vi "STAGE+mono+counter_edit25.vi"() -> ()   [LabVIEW 2017]
panel:
  out "Timeout":bool
  out "PROGRESS":u8(slide) max=10 step=10 scale=0.0..1.0
  in  "?":enum32{"Scan Data", "Scans", "RT Data"}(tab)
  out "Spectrum":cluster{dbl[], dbl[]}(graph)
  out "Decay":cluster{dbl[], dbl[]}[](graph)
  in  "Collect Data!":bool
  out "Waveform Graph":waveform(dbl)[](graph)
  out "?":i32(knob) scale=0.0..1000000.0
  out "Photon Counts":dbl
  in  "Wavelength":dbl
  in  "Show Real Time Data":bool
  in  "?":enum32{"DELAY", "COUNTER", "MONO", "PLOT"}(tab)
  in  "Data File Path":path
  out "Final time [ps]":dbl
  out "Current time [ps]":dbl
  out "Initial time [ps]":dbl
  in  "Set this as t0":bool
  in  "Axis":i32=1
  in  "Motor ON":bool
  in  "Motor OFF":bool
  out "Current Position [mm]":dbl
  out "Final Position [mm]":dbl
  in  "Data Points":i32=100
  out "Current Point":i32
  in  "Step Size [um]":i32=10
  in  "Target [mm]":dbl format="%.3f"
  in  "Move":bool
  out "Initial position [mm]":dbl
  in  "GPIB address":string="23"
  in  "Count Mode":u16(ring) items=["A,B for Preset T", "A-B for Preset T", "A+B for Preset T", "A for Preset B"]
  in  "Trigger mode":u16(ring) items=["10 MHz"=0, "Input 2"=2, "Input T"=3]
  in  "Channel A Input":u16(ring)=1 items=["10 MHz", "Input 1"]
  in  "Channel B Input":u16(ring)=2 items=["Input 1"=1, "Input 2"=2]
  in  "Number of Measurements\n to take at one point/ Number of Periods":u16=1 min=1 max=2000 step=1
  in  "Time between measurements\n at one point (s)/Dwell Time":dbl=0.002 min=0.002 max=60.0 step=0.001
  in  "gate mode (CW:0)":i16(slide) scale=0.0..2.0 scale format="%.2f"
  out "Counts":i32
  in  "Integrating time \nin 10^-7 sec":dbl=10000000.0
  in  "Discriminator Level (mV)":dbl min=-300.0 max=300.0 step=0.2
  in  "Discriminator Slope":bool
  in  "Channel":i16 min=0 max=2 step=1
  out "Grating #":dbl
  out "Blaze angle":dbl
  out "Grooves/mm":dbl
  out "Mono port":T1(ring)
  out "Time delay":u32=450000 min=1
  in  "Step size":dbl=10.0 min=0.0
  in  "Scan to":i32=4000
  in  "Scan from":i32=2600
  out "Current wavelength":dbl
  in  "?":bool
  in  "NEW UNIT":T2(ring)
  in  "Array":dbl[](array[numeric])
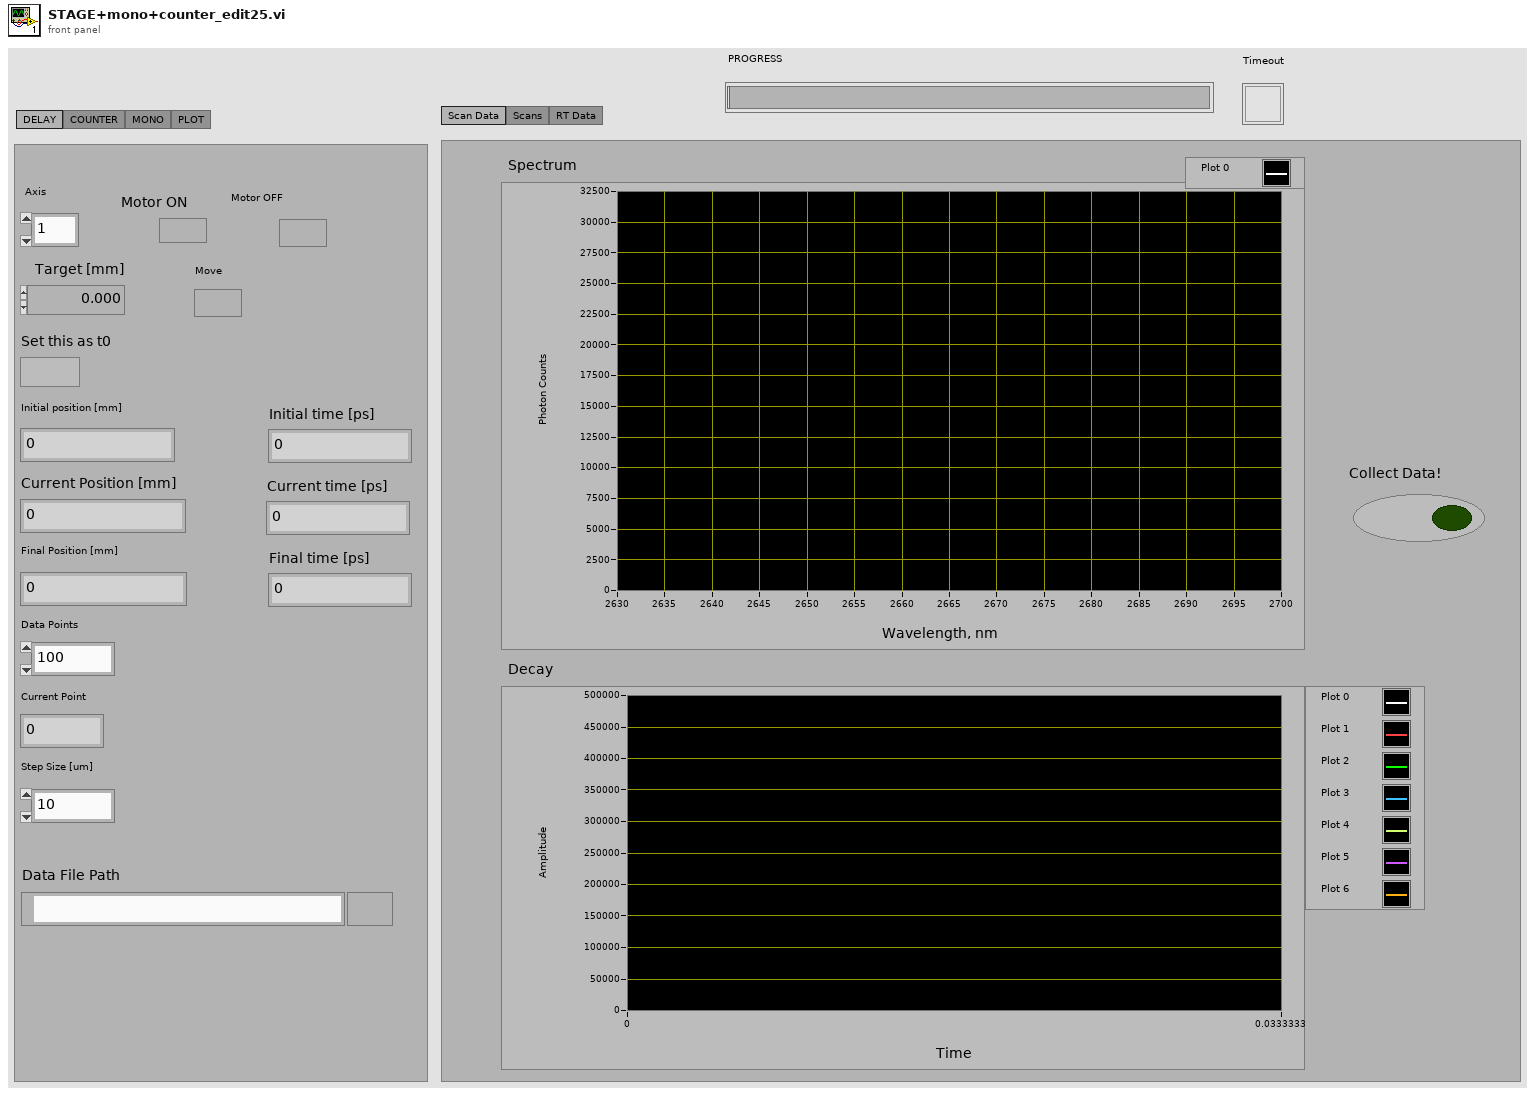
[diagram p1: front panel]
types:
  T1 = enum8{"COM 1", "COM 2", "COM 3", "COM 4", "COM 5", "COM 6", "COM 7", "COM 8", "COM 9"}
  T2 = enum16{"centi-Microns", " Nanometers", "   Angstroms"}
  T3 = cluster{"input XON/XOFF":bool, "input HW Handshake":bool, "input alt HW HShk":bool, "output XON/XOFF":bool, "output HW Handshake":bool, "output alt HW HShk":bool, "XOFF byte":u8, "XON byte":u8, "parity error byte":u16}
  T4 = enum16{"no parity", "odd parity", "even parity", "mark parity", "space parity"}
  T5 = enum16{"open", "replace", "create", "open or create", "replace or create", "replace or create with confirmation"}
  T6 = typedef "NI_Matrix.lvlib/RealMatrix.ctl" = dbl[][]
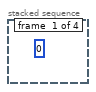
[diagram p2: hidden frame]
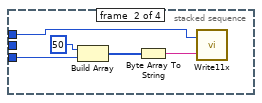
[diagram p3: hidden frame]
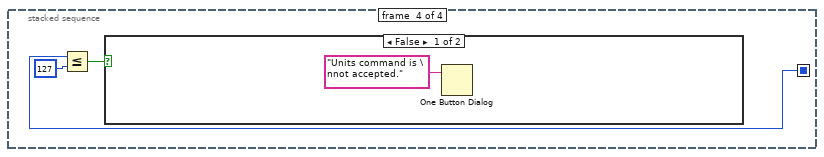
[diagram p4: hidden frame]
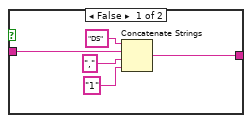
[diagram p7: hidden frame]
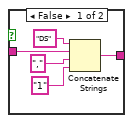
[diagram p9: hidden frame]
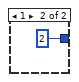
[diagram p13: hidden frame]
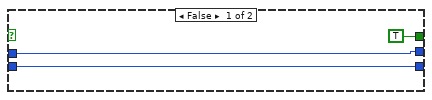
[diagram p14: hidden frame]
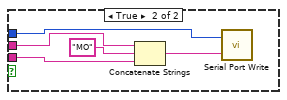
[diagram p15: hidden frame]
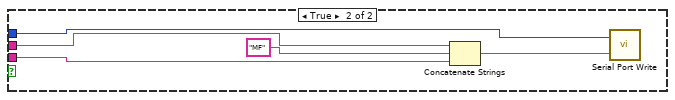
[diagram p16: hidden frame]
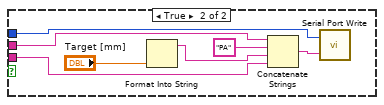
[diagram p17: hidden frame]
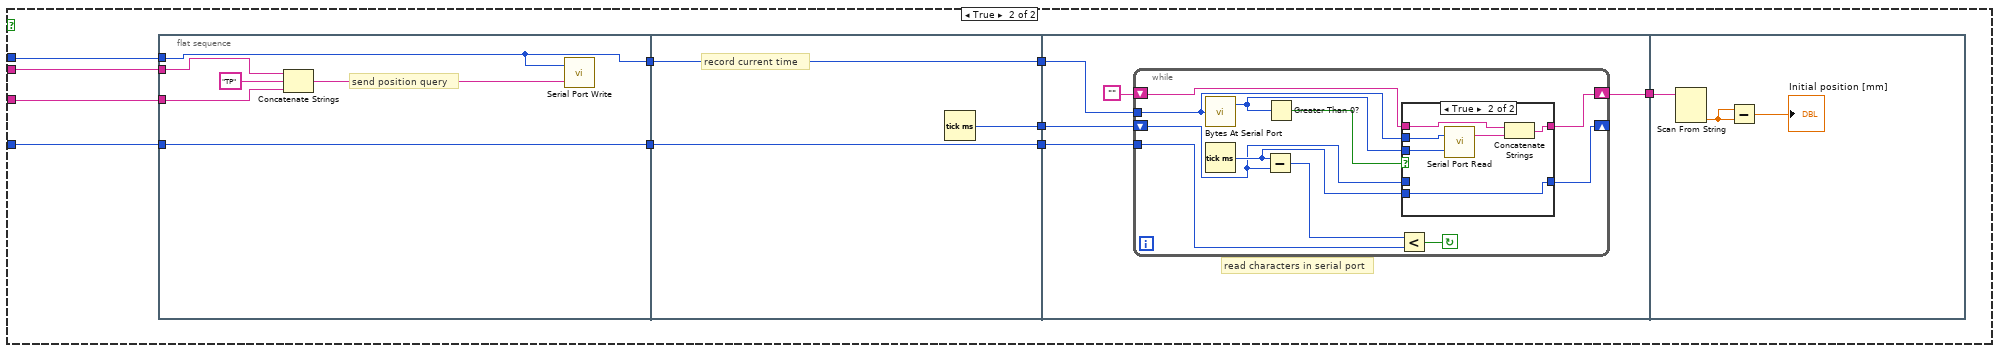
[diagram p18: hidden frame]
diagram:
  w29 = u32 19200  # baud rate
  w28 = u16 8  # data bits
  w27 = enum16{"1 bit", "1.5 bits", "2 bits"}."1 bit"  # stop bits
  w31 = T4."no parity"  # parity
  w9 = 4  # 0=COM1 so n=COM(n+1)
  w30 = u16 1024  # buffer size
  n1 = flat-sequence {
    tunnel: [w34] -> w1
    tunnel: [w33] -> w2
    frame #0 {
      n2 = call "CM Com Read ini.vi"() -> ("Mono port"=w33:T1, "time delay1"=w34:u32)  [unwired: 7 in]
    }
  }
  n3 = stacked-sequence {
    seq-local: [_ _ w42 _] -> [_ _ _ w49]
    tunnel: "NEW UNIT" -> [_ w36 _ _]
    tunnel: w1 -> [_ w35 w40 _]
    tunnel: w2 -> [_ _ w41 _]
    frame #0 {
      (unwired) u8 0
    }
    frame #1 {
      n4 = Build Array(u8 50, w36) -> (w38:u16[])
      n5 = Byte Array To String(unsigned byte array=w38) -> (string=w37:string)
      n6 = call "Write11x.vi"("string to write"=w37, "port number"=w35) -> ()  [unwired: 1 out]
    }
    frame #2 {
      n7 = call "Read11x.vi"("response size"=2, "timeout count"=w41, "port number"=w40) -> ("rcv index"=w43:u8[])  [unwired: 2 out]
      n8 = Index Array(array=w43, index=1) -> ()  [unwired: 1 out]
      n9 = Index Array(array=w43, index=0) -> (element=w42:u8)
    }
    frame #3 {
      n10 = Less Or Equal?(x=w49, y=127) -> (x <= y?=w47:bool)
      n11 = case shown="False" w47 {
        frame False {
          n12 = One Button Dialog(message="Units command is \nnot accepted.") -> ()  [unwired: 1 in, 1 out]
        }
        frame True {
        }
      }
    }
  }
  n13 = call "CM Serial Port Setup.vi"("COM port"=w2, "time delay"=w1) -> ("time delay1"=w19:u32, "DK port Out"=w20:T1, "error code"=w22:i32)  [unwired: 7 in]
  n14 = Equal To 0?(x=w22) -> (x = 0?=w21:bool)
  n15 = case shown="True" w21 {
    tunnel: w20 -> [w53 w56]
    tunnel: w19 -> [w52 w55]
    tunnel: [w53 w56] -> w6
    tunnel: [w52 w55] -> w5
    tunnel: [TRUE FALSE] -> w4
    frame False {
    }
    frame True {
      n16 = call "CM Com Write ini.vi"("time delay1"=w56, "Mono port"=w55) -> ()  [unwired: 7 in]
      n17 = local write "Mono port"(w56) -> ()
      n18 = local write "Time delay"(w55) -> ()
    }
  }
  n19 = call <vilib>:"Serial Port Init.vi"("flow control etc."=T3 {"input XON/XOFF"=FALSE, "input HW Handshake"=FALSE, "input alt HW HShk"=FALSE, "output XON/XOFF"=FALSE, "output HW Handshake"=FALSE, "output alt HW HShk"=FALSE, "XOFF byte"=13, "XON byte"=11, "parity error byte"=0}, "parity"=w31, "buffer size"=w30, "stop bits"=w27, "data bits"=w28, "baud rate"=w29, "port number"=w9) -> ("error code"=w26:i32)
  n20 = Concatenate Strings("\r", "\n") -> (w23:string)
  n21 = while {
    tunnel: w5 -> [w59]
    tunnel: w6 -> [w58]
    stop <- TRUE continue-if-true
    n22 = case shown="True" "?" {
      tunnel: w59 -> [_ w62]
      tunnel: w58 -> [_ w61]
      frame False {
      }
      frame True {
        n23 = Two Button Dialog(message="Do you want to change grating?", 1:"No" ("F button name (\"Cancel\")"), 2:"Yes" ("T button name (\"OK\")")) -> (T button?=w63:bool)
        n24 = case shown="True" w63 {
          tunnel: w62 -> [_ w68]
          tunnel: w61 -> [_ w67]
          frame False {
          }
          frame True {
            n25 = Two Button Dialog(message="Disable voltage from PMT", 1:"Do not swich grating" ("F button name (\"Cancel\")"), 2:"Done" ("T button name (\"OK\")")) -> (T button?=w69:bool)
            n26 = case shown="True" w69 {
              tunnel: w68 -> [_ w81]
              tunnel: w67 -> [_ w80]
              frame False {
              }
              frame True {
                n27 = flat-sequence {
                  tunnel: w81 -> [w85]
                  tunnel: [w85] -> w75
                  tunnel: w80 -> [w84]
                  tunnel: [w84] -> w74
                  tunnel: [w82] -> w73
                  tunnel: w75 -> [w90]
                  tunnel: [w90] -> w78
                  tunnel: w74 -> [w91]
                  tunnel: [w91] -> w77
                  tunnel: w73 -> [w89]
                  tunnel: [w89] -> w76
                  tunnel: w78 -> [w95]
                  tunnel: w77 -> [w96]
                  tunnel: [w94] -> w79
                  tunnel: w76 -> [w94]
                  frame #0 {
                    n28 = local read "Grating #"() -> (w83:dbl)
                    n29 = case shown="2, Default" w83 {
                      tunnel: [1 2] -> w82
                      frame 2, Default {
                      }
                      frame 1 {
                      }
                    }
                    n30 = call "Select11x2.vi"("time delay"=w85, "NEW GRT?"=w82, "port number"=w84) -> ()  [unwired: 3 out]
                  }
                  frame #1 {
                    n31 = call "Query11x.vi"("port number"=w91, "QUERY"=u16 2, "time delay"=w90) -> ("STATUS MESSAGE"=w88:u16)  [unwired: 3 out]
                    n32 = local write "Grooves/mm"(w88) -> ()
                  }
                  frame #2 {
                    n33 = Divide(x=w95, y=i16 100 ("device (1)")) -> (x/y=w97:dbl)
                    n34 = call "Query11x.vi"("port number"=w96, "QUERY"=u16 3, "time delay"=w97) -> ("STATUS MESSAGE"=w93:u16)  [unwired: 3 out]
                    n35 = local write "Blaze angle"(w93) -> ()
                  }
                }
                n36 = local write "Grating #"(w79) -> ()
              }
            }
          }
        }
      }
    }
  }
  n37 = while {
    tunnel: w9 -> [w114]
    tunnel: w23 -> [w115]
    tunnel: w26 -> [_]
    tunnel: "Axis" -> [w112]
    stop <- TRUE continue-if-true
    w113 = u32 200  # timeout
    n38 = Format Into String(w112) -> (resulting string=w116:string)  [unwired: 3 in, 1 out]
    n39 = flat-sequence {
      tunnel: w116 -> [w121]
      tunnel: w115 -> [w120]
      tunnel: w114 -> [w122]
      tunnel: w113 -> [w119]
      tunnel: [w121] -> w111
      tunnel: [w120] -> w110
      tunnel: [w122] -> w109
      tunnel: [w119] -> w108
      tunnel: w111 -> [w132]
      tunnel: w110 -> [w131]
      tunnel: w109 -> [w133]
      tunnel: w108 -> [w129]
      tunnel: [w132] -> w107
      tunnel: [w131] -> w106
      tunnel: [w133] -> w105
      tunnel: [w129] -> w104
      tunnel: w107 -> [w142]
      tunnel: w106 -> [w141]
      tunnel: w105 -> [w143]
      tunnel: w104 -> [w139]
      tunnel: [w142] -> w103
      tunnel: [w141] -> w102
      tunnel: [w143] -> w101
      tunnel: [w139] -> w100
      tunnel: w103 -> [w155]
      tunnel: w102 -> [w152]
      tunnel: w101 -> [w154]
      tunnel: w100 -> [w153]
      frame #0 {
        n40 = case shown="False" "Motor ON" {
          tunnel: w122 -> [_ w128]
          tunnel: w121 -> [_ w125]
          tunnel: w120 -> [_ w124]
          frame False {
          }
          frame True {
            n41 = Concatenate Strings(w125, "MO" ("Substring"), w124) -> (w126:string)
            n42 = call <vilib>:"Serial Port Write.vi"("string to write"=w126, "port number"=w128) -> ()  [unwired: 1 out]
          }
        }
      }
      frame #1 {
        n43 = case shown="False" "Motor OFF" {
          tunnel: w133 -> [_ w138]
          tunnel: w132 -> [_ w135]
          tunnel: w131 -> [_ w134]
          frame False {
          }
          frame True {
            n44 = Concatenate Strings(w135, "MF" ("Substring"), w134) -> (w136:string)
            n45 = call <vilib>:"Serial Port Write.vi"("string to write"=w136, "port number"=w138) -> ()  [unwired: 1 out]
          }
        }
      }
      frame #2 {
        n46 = case shown="False" "Move" {
          tunnel: w143 -> [_ w150]
          tunnel: w142 -> [_ w147]
          tunnel: w141 -> [_ w146]
          frame False {
          }
          frame True {
            n47 = Format Into String("Target [mm]") -> (resulting string=w144:string)  [unwired: 3 in, 1 out]
            n48 = Concatenate Strings(w147, "PA" ("Substring"), w144, w146) -> (w148:string)
            n49 = call <vilib>:"Serial Port Write.vi"("string to write"=w148, "port number"=w150) -> ()  [unwired: 1 out]
          }
        }
      }
      frame #3 {
        n50 = case shown="False" "Set this as t0" {
          tunnel: w155 -> [_ w165]
          tunnel: w154 -> [_ w164]
          tunnel: w153 -> [_ w163]
          tunnel: w152 -> [_ w162]
          frame False {
          }
          frame True {
            n51 = flat-sequence {
              tunnel: w165 -> [w169]
              tunnel: w164 -> [w168]
              tunnel: [w168] -> w161
              tunnel: w163 -> [w166]
              tunnel: [w166] -> w160
              tunnel: w162 -> [w167]
              tunnel: w161 -> [w173]
              tunnel: [w173] -> w159
              tunnel: w160 -> [w172]
              tunnel: [w172] -> w158
              tunnel: [w174] -> w157
              tunnel: w159 -> [w179]
              tunnel: w158 -> [w177]
              tunnel: w157 -> [w176]
              tunnel: [w175] -> w156
              tunnel: w156 -> [w201]
              frame #0 {
                # "send position query"
                n52 = Concatenate Strings(w169, "TP" ("Substring"), w167) -> (w170:string)
                n53 = call <vilib>:"Serial Port Write.vi"("string to write"=w170, "port number"=w168) -> ()  [unwired: 1 out]
              }
              frame #1 {
                # "record current time"
                n54 = Tick Count (ms)() -> (millisecond timer value=w174:u32)
              }
              frame #2 {
                # "read characters in serial port"
                n55 = while {
                  shift-left: w176 -> [w180]
                  shift-right: [w181] -> _
                  tunnel: w177 -> [w184]
                  shift-left: "" -> [w187]
                  shift-right: [w186] -> w175
                  tunnel: w179 -> [w188]
                  stop <- w183 continue-if-true
                  n56 = call <vilib>:"Bytes At Serial Port.vi"("port number"=w188) -> ("byte count"=w189:u32)  [unwired: 1 out]
                  n57 = Tick Count (ms)() -> (millisecond timer value=w182:u32)
                  n58 = Subtract(x=w182, y=w180) -> (x-y=w185:u32)
                  n59 = Greater Than 0?(x=w189) -> (x > 0?=w190:bool)
                  n60 = Less?(x=w185, y=w184) -> (x < y?=w183:bool)
                  n61 = case shown="True" w190 {
                    tunnel: w189 -> [_ w198]
                    tunnel: w188 -> [_ w197]
                    tunnel: w187 -> [w192 w195]
                    tunnel: [w192 w194] -> w186
                    tunnel: [w191 w193] -> w181
                    tunnel: w182 -> [_ w193]
                    tunnel: w180 -> [w191 _]
                    frame False {
                    }
                    frame True {
                      n62 = call <vilib>:"Serial Port Read.vi"("requested byte count"=w198, "port number"=w197) -> ("string read"=w196:string)  [unwired: 1 out]
                      n63 = Concatenate Strings(w195, w196) -> (w194:string)
                    }
                  }
                }
              }
              frame #3 {
                n64 = Scan From String(input string=w201) -> (output 1=w199:dbl)  [unwired: 4 in, 3 out]
                n65 = Subtract(x=w199, y=w199) -> (x-y=→"Initial position [mm]":dbl)
              }
            }
          }
        }
      }
    }
    n66 = Wait Until Next ms Multiple(millisecond multiple=u32 50) -> ()  [unwired: 1 out]
  }
  n67 = while {
    tunnel: "GPIB address" -> [w205]
    tunnel: w6 -> [w204]
    tunnel: w5 -> [w203]
    tunnel: w4 -> [w202]
    stop <- TRUE continue-if-true
    n68 = case shown="True" "Show Real Time Data" {
      tunnel: w205 -> [_ w214]
      tunnel: w204 -> [_ w211]
      tunnel: w203 -> [_ w208]
      tunnel: w202 -> [_ w213]
      frame False {
      }
      frame True {
        n69 = flat-sequence {
          tunnel: w214 -> [w243]
          tunnel: "Wavelength" -> [w244]
          tunnel: [w244] -> w225
          tunnel: [w233] -> w224
          tunnel: [w234] -> w223
          tunnel: [w243] -> w222
          tunnel: w208 -> [w234]
          tunnel: w211 -> [w233]
          tunnel: w213 -> [_]
          tunnel: [w232] -> w209
          tunnel: w208 -> [w232]
          tunnel: [w252] -> w221
          tunnel: [w251] -> w220
          tunnel: [w249] -> w219
          tunnel: w225 -> [w247]
          tunnel: w224 -> [w252]
          tunnel: w223 -> [w251]
          tunnel: w222 -> [w249]
          tunnel: [w245] -> w210
          tunnel: w209 -> [w245]
          tunnel: w221 -> [_]
          tunnel: w220 -> [_]
          tunnel: w219 -> [w255]
          tunnel: [w255] -> w218
          tunnel: w211 -> [w254]
          tunnel: w210 -> [w253]
          tunnel: w218 -> [w264]
          tunnel: [w264] -> w217
          tunnel: w217 -> [w314]
          tunnel: [w314] -> w216
          tunnel: w216 -> [w315]
          tunnel: [w315] -> w215
          tunnel: w215 -> [w325]
          frame #0 {
            n70 = call "Query11x.vi"("port number"=w233, "QUERY"=u16 0, "time delay"=w234) -> ("timeout"=w230:bool, "STATUS MESSAGE"=w229:u16)  [unwired: 2 out]
            n71 = call "Query11x.vi"("port number"=w233, "QUERY"=u16 2, "time delay"=w234) -> ("timeout"=w241:bool, "STATUS MESSAGE"=w240:u16)  [unwired: 2 out]
            n72 = call "Query11x.vi"("port number"=w233, "QUERY"=u16 4, "time delay"=w234) -> ("timeout"=w235:bool, "STATUS MESSAGE"=w236:u16)  [unwired: 2 out]
            n73 = call "Query11x.vi"("port number"=w233, "QUERY"=u16 3, "time delay"=w234) -> ("timeout"=→"Timeout":bool, "STATUS MESSAGE"=w238:u16)  [unwired: 2 out]
            n74 = local write "Timeout"(w230) -> ()
            n75 = local write "Timeout"(w241) -> ()
            n76 = local write "Grooves/mm"(w240) -> ()
            n77 = local write "Timeout"(w235) -> ()
            n78 = local write "Grating #"(w236) -> ()
            n79 = Divide(x=w229, y=10 ("Numeric")) -> (x/y=w227:dbl)
            n80 = local write "Current wavelength"(w227) -> ()
            n81 = local write "Blaze angle"(w238) -> ()
          }
          frame #1 {
            n82 = Multiply(x=w247, y=1) -> (x*y=w246:dbl)
            n83 = call "Goto11x.vi"("time delay"=w251, "WAVELENGTH"=w246, "port number"=w252) -> ("timeout"=w250:bool)  [unwired: 2 out]
            n84 = local write "Timeout"(w250) -> ()
          }
          frame #2 {
            # "set counter time in 10^-7 seconds in CW"
            n85 = call "Query11x.vi"("port number"=w254, "QUERY"=0, "time delay"=w253) -> ("timeout"=w259:bool, "STATUS MESSAGE"=w258:u16)  [unwired: 2 out]
            n86 = local write "Timeout"(w259) -> ()
            n87 = Divide(x=w258, y=1) -> (x/y=w257:dbl)
            n88 = local write "Current wavelength"(w257) -> ()
          }
          frame #3 {
            # "Configures discriminator."
            n89 = flat-sequence {
              tunnel: w264 -> [w271]
              tunnel: [w271] -> w270
              tunnel: [w278] -> w269
              tunnel: [w276] -> w268
              tunnel: w263 -> [w277]
              tunnel: w270 -> [w276]
              tunnel: w265 -> [w275]
              tunnel: w269 -> [w297]
              tunnel: [w298] -> w267
              tunnel: w268 -> [w296]
              tunnel: [w296] -> w266
              tunnel: w265 -> [w294]
              tunnel: w267 -> [w310]
              tunnel: w266 -> [w309]
              tunnel: w261 -> [w304]
              tunnel: w265 -> [w303]
              frame #0 {
                # "Flush I/O buffers."
                n90 = for {
                  N: 5 -> [_]
                  tunnel: w271 -> [w273]
                  n91 = GPIB Write(0:w273, 1:"\r") -> ()  [unwired: 3 in, 2 out]
                }
              }
              frame #1 {
                # "Set discriminator slope."
                n92 = case shown="True" w277 {
                  tunnel: [w284 w289] -> w279
                  tunnel: w275 -> [w283 w288]
                  frame False {
                    n93 = Concatenate Strings("DS", w283, ",", "1") -> (w284:string)
                  }
                  frame True {
                    n94 = Concatenate Strings("DS", w288, ",", "0") -> (w289:string)
                  }
                }
                n95 = GPIB Write(0:w276, 1:w279, 2:5) -> (6:w278:errorcluster)  [unwired: 2 in, 1 out]
              }
              frame #2 {
                # "Set discriminator mode to fixed."
                n96 = Concatenate Strings("DM", w294, ",", "0") -> (w293:string)
                n97 = GPIB Write(0:w296, 1:w293, 2:5, 3:w297) -> (6:w298:errorcluster)  [unwired: 1 in, 1 out]
              }
              frame #3 {
                # "Set discriminator level.\nMust be between +300 and -300 mV."
                n98 = Divide(x=w304, y=1000.0) -> (x/y=w312:dbl)
                n99 = Number To Fractional String(number=w312, precision (6)=i16 4) -> (F-format string=w301:string)  [unwired: 2 in]
                n100 = Concatenate Strings("DL", w303, ",", w301) -> (w308:string)
                n101 = GPIB Write(0:w309, 1:w308, 2:5, 3:w310) -> (6:w305:errorcluster)  [unwired: 1 in, 1 out]
                n102 = call <vilib>:"General Error Handler.vi"("type of dialog (OK msg:1)"=1, "error in (no error)"=w305) -> ()  [unwired: 9 in, 5 out]
              }
            }
            n103 = local read "Channel"() -> (w262:i16)
            n104 = local read "Discriminator Slope"() -> (w263:bool)
            n105 = Number To Decimal String(number=w262) -> (decimal integer string=w265:string)  [unwired: 1 in]
            n106 = local read "Discriminator Level (mV)"() -> (w261:dbl)
          }
          frame #4 {
            n107 = call "Start.vi"("GPIB Address"=w314) -> ()  [unwired: 9 in]
          }
          frame #5 {
            # "Wait for Scan to Finish"
            n108 = for {
              N: 1 -> [_]
              tunnel: w315 -> [w317]
              n109 = while {
                tunnel: w317 -> [w318]
                stop <- w320 stop-if-true
                n110 = call "ScanDone.vi"("Wait (ms)"=1000, "GPIB Address"=w318) -> ("Scan Finished?"=w320:bool)
              }
            }
          }
          frame #6 {
            n111 = call "Read Data.vi"("Channel Number"=0, "GPIB Address"=w325, "Number of Datapoints"=1) -> ("Data"=w326:i32[])
            n112 = property class="Knob (strict)"("Scale.Increment"=1000, "Scale.Maximum"=1000000, "Scale.Minimum"=0) -> ()  [unwired: 2 in, 2 out]
            n113 = Index Array(array=w326, index=0) -> (element=→"Photon Counts" →"?":i32)
          }
        }
      }
    }
  }
  n114 = while {
    tunnel: "Axis" -> [w338]
    tunnel: w9 -> [w337]
    tunnel: "GPIB address" -> [w336]
    tunnel: "Integrating time \nin 10^-7 sec" -> [w335]
    tunnel: w5 -> [w334]
    tunnel: w6 -> [w333]
    tunnel: w4 -> [w332]
    stop <- TRUE continue-if-true
    n115 = case shown="True" "Collect Data!" {
      selector: "Collect Data!" -> [_ w339]
      tunnel: w338 -> [_ w347]
      tunnel: w337 -> [_ w346]
      tunnel: w336 -> [_ w345]
      tunnel: w336 -> [_ w343]
      tunnel: w335 -> [_ w342]
      tunnel: w334 -> [_ w341]
      tunnel: w333 -> [_ w344]
      tunnel: w332 -> [_ w340]
      frame False {
      }
      frame True {
        n116 = flat-sequence {
          tunnel: w347 -> [w367]
          tunnel: w346 -> [w365]
          tunnel: w345 -> [w364]
          tunnel: w344 -> [w363]
          tunnel: w343 -> [w362]
          tunnel: w342 -> [w359]
          tunnel: w341 -> [w352]
          tunnel: w340 -> [w351]
          tunnel: w339 -> [_]
          frame #0 {
            w372 = 1000000000000.0
            w377 = 1000
            w378 = 300000000
            w384 = 1
            n117 = Multiply(x="Step Size [um]", y="Data Points") -> (x*y=w381:i32)
            n118 = Divide(x="Step Size [um]", y=1000.0) -> (x/y=w390:dbl)
            n119 = local read "Initial position [mm]"() -> (w369:dbl)
            n120 = Multiply(x="Scan to", y=w384) -> (x*y=w358:i32)
            n121 = Increment(x="Data Points") -> (x+1=w399:i32)
            n122 = Multiply(x="Scan from", y=w384) -> (x*y=w357:i32)
            n123 = Divide(x=w381, y=1000) -> (x/y=w380:dbl)
            n124 = To Time Stamp(1:w357) -> (0:w387:timestamp)
            n125 = Multiply(x=w358, y=1) -> (x*y=w396:i32)
            n126 = Multiply(x=1, y=w357) -> (x*y=w361:i32)
            n127 = Divide(x=w390, y=1000.0) -> (x/y=w391:dbl)
            n128 = for {
              N: w399 -> [_]
              tunnel: w390 -> [w764]
              tunnel: w369 -> [w762]
              tunnel: [w755] -> w398 mode=indexing
              i -> [w763]
              # "distances"
              n129 = Multiply(x=w764, y=w763) -> (x*y=w761:dbl)
              n130 = Add(x=w762, y=w761) -> (x+y=w760:dbl)
              n131 = Divide(x=w760, y=1000) -> (x/y=w754:dbl)
              n132 = Divide(x=w754, y=300000000) -> (x/y=w757:dbl)
              n133 = Multiply(x=w757, y=1000000000000.0) -> (x*y=w755:dbl)
            }
            n134 = Subtract(x=w396, y=w361) -> (x-y=w402:i32)
            n135 = Divide(x=w369, y=w377) -> (x/y=w375:dbl)
            n136 = Add(x=w369, y=w380) -> (x+y=w371:dbl)
            "Final Position [mm]" <- w371
            n137 = property on="Waveform Graph" class="WFGraph (strict)"("XScale.Increment"="Step size", "XScale.Maximum"=w358, "XScale.Minimum"=w357) -> ()  [unwired: 2 in, 2 out]
            n138 = Divide(x=w371, y=w377) -> (x/y=w376:dbl)
            n139 = Divide(x=w402, y="Step size") -> (x/y=w401:dbl)
            n140 = Divide(x=w375, y=w378) -> (x/y=w374:dbl)
            n141 = Divide(x=w391, y=300000000) -> (x/y=w393:dbl)
            n142 = Bundle By Name("Y"=dbl[] [], "t0"=w387, "dt"="Step size") -> (w386:waveform(dbl))  [unwired: 1 in]
            n143 = Divide(x=w376, y=w378) -> (x/y=w373:dbl)
            n144 = Multiply(x=w393, y=1000000000000.0) -> (x*y=w355:dbl)
            n145 = Multiply(x=w374, y=w372) -> (x*y=w354:dbl)
            "Initial time [ps]" <- w354
            n146 = Round Toward -Infinity(1:w401) -> (0:w360:dbl)
            n147 = Concatenate Strings("\r", "\n") -> (w366:string)
            n148 = Build Array(w386) -> (w350:waveform(dbl)[])
            n149 = Multiply(x=w373, y=w372) -> (x*y=w385:dbl)
            "Final time [ps]" <- w385
            n150 = Increment(x=w360) -> (x+1=w389:dbl)
            n151 = for {
              N: w389 -> [_]
              tunnel: "Step size" -> [w769]
              tunnel: w361 -> [w767]
              tunnel: [w765] -> _ mode=indexing
              i -> [w768]
              # "wavelengths"
              n152 = Multiply(x=w769, y=w768) -> (x*y=w766:dbl)
              n153 = Add(x=w767, y=w766) -> (x+y=w765:dbl)
            }
            n154 = for {
              N: "Data Points" -> [w426]
              tunnel: w369 -> [w467]
              tunnel: "Step Size [um]" -> [w463]
              tunnel: w367 -> [w460]
              tunnel: w366 -> [w457]
              tunnel: w365 -> [w458]
              tunnel: w364 -> [w456]
              tunnel: w363 -> [w454]
              tunnel: w362 -> [w455]
              tunnel: w361 -> [w417]
              tunnel: "Step size" -> [w449]
              tunnel: w360 -> [w448]
              tunnel: w359 -> [w447]
              tunnel: w358 -> [w412]
              tunnel: w357 -> [w411]
              tunnel: "Step size" -> [w413]
              tunnel: w355 -> [w428]
              tunnel: w354 -> [w445]
              shift-right: [w427] -> _
              shift-left: dbl[] [] -> [w423]
              tunnel: w352 -> [w440]
              tunnel: w363 -> [w439]
              tunnel: w351 -> [w438]
              shift-right: [w433] -> _
              shift-left: w350 -> [w434]
              shift-right: [w421] -> _
              shift-left: dbl[][] [] -> [w420]
              shift-right: [w409] -> _
              shift-left: dbl[][] [] -> [w407]
              i -> [w415]
              w437 = dbl[] []
              n155 = stacked-sequence {
                tunnel: w454 -> [w737]
                tunnel: w455 -> [_]
                frame #0 {
                  n156 = call <vilib>:"Close Serial Driver.vi"("port number"=w737) -> ()  [unwired: 1 out]
                  n157 = GPIB Misc(0:"loc 23" ("command string")) -> ()  [unwired: 1 in, 3 out]
                }
              }
              n158 = property on="Waveform Graph" class="WFGraph (strict)"("XScale.Increment"=w413, "XScale.Maximum"=w412, "XScale.Minimum"=w411) -> ()  [unwired: 2 in, 2 out]
              n159 = Number To Decimal String(number=w447) -> (decimal integer string=w452:string)  [unwired: 1 in]
              n160 = Divide(x=w463, y=1000) -> (x/y=w462:dbl)
              n161 = property on="PROGRESS" class="Slide (strict)"("Scale.Increment"=1, "Scale.Maximum"=w426, "Scale.Minimum"=0) -> ()  [unwired: 2 in, 2 out]
              n162 = Multiply(x=w428, y=w415) -> (x*y=w446:dbl)
              n163 = Add(x=1, y=w415) -> (x+y=→"PROGRESS":i32)
              n164 = Concatenate Strings("CP 2,", w452) -> (w450:string)
              n165 = Add(x=w445, y=w446) -> (x+y=w424:dbl)
              n166 = Multiply(x=w462, y=w415) -> (x*y=w466:dbl)
              n167 = Add(x=w467, y=w466) -> (x+y=w465:dbl)
              n168 = Build Array (concatenate)(w423, w424) -> (w425:dbl[])
              n169 = Format Into String(w460) -> (resulting string=w459:string)  [unwired: 3 in, 1 out]
              n170 = GPIB Write(0:w456, 1:w450, 2:i16 5 ("mode (0)")) -> ()  [unwired: 2 in, 2 out]
              n171 = flat-sequence {
                tunnel: w465 -> [w740]
                tunnel: [w740] -> w461
                tunnel: w457 -> [w742]
                tunnel: w459 -> [w741]
                tunnel: w458 -> [w738]
                tunnel: w461 -> [w751]
                tunnel: [w746] -> w410
                frame #0 {
                  n172 = Format Into String(w740) -> (resulting string=w739:string)  [unwired: 3 in, 1 out]
                  n173 = Wait (ms)(milliseconds to wait=u32 100) -> ()  [unwired: 1 out]
                  n174 = Concatenate Strings(w741, "PA" ("Substring"), w739, w742) -> (w744:string)
                  n175 = call <vilib>:"Serial Port Write.vi"("string to write"=w744, "port number"=w738) -> ()  [unwired: 1 out]
                }
                frame #1 {
                  n176 = Divide(x=w751, y=1000) -> (x/y=w749:dbl)
                  n177 = Wait (ms)(milliseconds to wait=u32 1000) -> ()  [unwired: 1 out]
                  n178 = Divide(x=w749, y=300000000) -> (x/y=w748:dbl)
                  n179 = Multiply(x=w748, y=1000000000000.0) -> (x*y=w746:dbl)
                  "Current time [ps]" <- w746
                  "Current Position [mm]" <- w751
                }
              }
              n180 = Add(x=w415, y=1) -> (x+y=w414:i32)
              n181 = flat-sequence {
                tunnel: w456 -> [w493]
                tunnel: w417 -> [w492]
                tunnel: w449 -> [w491]
                tunnel: w448 -> [w490]
                tunnel: w412 -> [w489]
                tunnel: w411 -> [w488]
                tunnel: w437 -> [w487]
                tunnel: w437 -> [w486]
                tunnel: w413 -> [w485]
                tunnel: w440 -> [w484]
                tunnel: w439 -> [w483]
                tunnel: w438 -> [w482]
                tunnel: [w480] -> w436
                tunnel: [w481] -> _
                tunnel: [w480] -> w435
                tunnel: w414 -> [w479]
                tunnel: w410 -> [w478]
                tunnel: [w477] -> w408
                tunnel: w407 -> [w476]
                tunnel: w436 -> [w715]
                tunnel: [w718] -> w422
                tunnel: [w717] -> w419
                tunnel: [w716] -> w409
                tunnel: w408 -> [w716]
                frame #0 {
                  # "step size"
                  n182 = while {
                    tunnel: w493 -> [w535]
                    tunnel: w492 -> [w556]
                    tunnel: w491 -> [w528]
                    tunnel: w490 -> [w555]
                    tunnel: w489 -> [w531]
                    tunnel: w488 -> [w530]
                    tunnel: w485 -> [w532]
                    shift-right: [w552] -> w480
                    shift-left: w486 -> [w551]
                    shift-right: [w547] -> w481
                    shift-left: w487 -> [w554]
                    tunnel: w484 -> [w494]
                    tunnel: w483 -> [w495]
                    tunnel: w482 -> [w537]
                    tunnel: w479 -> [w516]
                    tunnel: w478 -> [w504]
                    shift-right: [w497] -> w477
                    shift-left: w476 -> [w496]
                    i -> [w524]
                    stop <- w526 stop-if-true
                    n183 = property on="Spectrum" class="XYGraph (strict)"("XScale.Increment"=w532, "XScale.Maximum"=w531, "XScale.Minimum"=w530) -> ()  [unwired: 2 in, 2 out]
                    n184 = Multiply(x=1, y=w528) -> (x*y=w527:dbl)
                    n185 = Multiply(x=w524, y=w527) -> (x*y=w557:dbl)
                    n186 = Greater Or Equal?(x=w524, y=w555) -> (x >= y?=w526:bool)
                    n187 = Add(x=w557, y=w556) -> (x+y=w536:dbl)
                    n188 = Add(x=w524, y=1) -> (x+y=w517:i32)
                    n189 = Build Array (concatenate)(w554, w536) -> (w553:dbl[])
                    n190 = flat-sequence {
                      tunnel: w535 -> [w577]
                      tunnel: w536 -> [w578]
                      tunnel: [w578] -> w541
                      tunnel: [w559] -> w540
                      tunnel: [w558] -> w539
                      tunnel: [w577] -> w538
                      tunnel: w494 -> [w558]
                      tunnel: w495 -> [w559]
                      tunnel: w537 -> [_]
                      tunnel: [w576] -> w518
                      tunnel: w517 -> [w576]
                      tunnel: [w575] -> w505
                      tunnel: w504 -> [w575]
                      tunnel: w496 -> [w574]
                      tunnel: [w574] -> w503
                      tunnel: [w588] -> w546
                      tunnel: [w587] -> w545
                      tunnel: [w585] -> w544
                      tunnel: w541 -> [w581]
                      tunnel: w540 -> [w588]
                      tunnel: w539 -> [w587]
                      tunnel: w538 -> [w585]
                      tunnel: [w582] -> w519
                      tunnel: w518 -> [w582]
                      tunnel: [w581] -> w511
                      tunnel: [w580] -> w506
                      tunnel: w505 -> [w580]
                      tunnel: w503 -> [w579]
                      tunnel: [w579] -> w502
                      tunnel: w546 -> [_]
                      tunnel: w545 -> [_]
                      tunnel: w544 -> [w595]
                      tunnel: [w595] -> w534
                      tunnel: [w594] -> w520
                      tunnel: w519 -> [w594]
                      tunnel: [w593] -> w512
                      tunnel: w511 -> [w593]
                      tunnel: [w592] -> w507
                      tunnel: w506 -> [w592]
                      tunnel: w502 -> [w591]
                      tunnel: [w591] -> w501
                      tunnel: w495 -> [w590]
                      tunnel: w494 -> [w589]
                      tunnel: w534 -> [w605]
                      tunnel: [w605] -> w533
                      tunnel: [w604] -> w521
                      tunnel: w520 -> [w604]
                      tunnel: [w603] -> w513
                      tunnel: w512 -> [w603]
                      tunnel: [w602] -> w508
                      tunnel: w507 -> [w602]
                      tunnel: w501 -> [w601]
                      tunnel: [w601] -> w500
                      tunnel: w533 -> [w662]
                      tunnel: [w662] -> w543
                      tunnel: [w661] -> w522
                      tunnel: w521 -> [w661]
                      tunnel: [w660] -> w514
                      tunnel: w513 -> [w660]
                      tunnel: [w659] -> w509
                      tunnel: w508 -> [w659]
                      tunnel: w500 -> [w658]
                      tunnel: [w658] -> w499
                      tunnel: w543 -> [w667]
                      tunnel: [w667] -> w542
                      tunnel: [w666] -> w523
                      tunnel: w522 -> [w666]
                      tunnel: [w665] -> w515
                      tunnel: w514 -> [w665]
                      tunnel: [w664] -> w510
                      tunnel: w509 -> [w664]
                      tunnel: w499 -> [w663]
                      tunnel: [w663] -> w498
                      tunnel: [w678] -> w549
                      tunnel: w542 -> [w710]
                      tunnel: w523 -> [w676]
                      tunnel: w516 -> [w679]
                      tunnel: w515 -> [w680]
                      tunnel: w510 -> [w682]
                      tunnel: w498 -> [w677]
                      tunnel: [w675] -> w497
                      frame #0 {
                        n191 = call "Query11x.vi"("port number"=w559, "QUERY"=u16 2, "time delay"=w558) -> ("timeout"=w567:bool, "STATUS MESSAGE"=→"Grooves/mm":u16)  [unwired: 2 out]
                        n192 = call "Query11x.vi"("port number"=w559, "QUERY"=u16 0, "time delay"=w558) -> ("timeout"=w572:bool, "STATUS MESSAGE"=w571:u16)  [unwired: 2 out]
                        n193 = call "Query11x.vi"("port number"=w559, "QUERY"=u16 3, "time delay"=w558) -> ("timeout"=w564:bool, "STATUS MESSAGE"=→"Blaze angle":u16)  [unwired: 2 out]
                        n194 = call "Query11x.vi"("port number"=w559, "QUERY"=u16 4, "time delay"=w558) -> ("timeout"=w561:bool, "STATUS MESSAGE"=→"Grating #":u16)  [unwired: 2 out]
                        n195 = local write "Timeout"(w572) -> ()
                        n196 = Divide(x=w571, y=1 ("Numeric")) -> (x/y=→"Current wavelength":dbl)
                        n197 = local write "Timeout"(w567) -> ()
                        n198 = local write "Timeout"(w564) -> ()
                        n199 = local write "Timeout"(w561) -> ()
                      }
                      frame #1 {
                        n200 = Multiply(x=w581, y=1) -> (x*y=w583:dbl)
                        n201 = call "Goto11x.vi"("time delay"=w587, "WAVELENGTH"=w583, "port number"=w588) -> ("timeout"=w586:bool)  [unwired: 2 out]
                        n202 = local write "Timeout"(w586) -> ()
                      }
                      frame #2 {
                        # "set counter time in 10^-7 seconds in CW"
                        n203 = call "Query11x.vi"("port number"=w590, "QUERY"=0, "time delay"=w589) -> ("timeout"=w599:bool, "STATUS MESSAGE"=w598:u16)  [unwired: 2 out]
                        n204 = local write "Timeout"(w599) -> ()
                        n205 = Divide(x=w598, y=1) -> (x/y=w597:dbl)
                        n206 = local write "Current wavelength"(w597) -> ()
                      }
                      frame #3 {
                        # "Configures discriminator."
                        n207 = flat-sequence {
                          tunnel: w605 -> [w615]
                          tunnel: [w615] -> w614
                          tunnel: [w622] -> w613
                          tunnel: [w620] -> w612
                          tunnel: "Discriminator Slope" -> [w621]
                          tunnel: w614 -> [w620]
                          tunnel: w606 -> [w619]
                          tunnel: w613 -> [w641]
                          tunnel: [w642] -> w611
                          tunnel: w612 -> [w640]
                          tunnel: [w640] -> w610
                          tunnel: w606 -> [w638]
                          tunnel: w611 -> [w654]
                          tunnel: w610 -> [w653]
                          tunnel: "Discriminator Level (mV)" -> [w648]
                          tunnel: w606 -> [w647]
                          frame #0 {
                            # "Flush I/O buffers."
                            n208 = for {
                              N: 5 -> [_]
                              tunnel: w615 -> [w617]
                              n209 = GPIB Write(0:w617, 1:"\r") -> ()  [unwired: 3 in, 2 out]
                            }
                          }
                          frame #1 {
                            # "Set discriminator slope."
                            n210 = case shown="True" w621 {
                              tunnel: [w628 w633] -> w623
                              tunnel: w619 -> [w627 w632]
                              frame False {
                                n211 = Concatenate Strings("DS", w627, ",", "1") -> (w628:string)
                              }
                              frame True {
                                n212 = Concatenate Strings("DS", w632, ",", "0") -> (w633:string)
                              }
                            }
                            n213 = GPIB Write(0:w620, 1:w623, 2:5) -> (6:w622:errorcluster)  [unwired: 2 in, 1 out]
                          }
                          frame #2 {
                            # "Set discriminator mode to fixed."
                            n214 = Concatenate Strings("DM", w638, ",", "0") -> (w637:string)
                            n215 = GPIB Write(0:w640, 1:w637, 2:5, 3:w641) -> (6:w642:errorcluster)  [unwired: 1 in, 1 out]
                          }
                          frame #3 {
                            # "Set discriminator level.\nMust be between +300 and -300 mV."
                            n216 = Divide(x=w648, y=1000.0) -> (x/y=w656:dbl)
                            n217 = Number To Fractional String(number=w656, precision (6)=i16 4) -> (F-format string=w645:string)  [unwired: 2 in]
                            n218 = Concatenate Strings("DL", w647, ",", w645) -> (w652:string)
                            n219 = GPIB Write(0:w653, 1:w652, 2:5, 3:w654) -> (6:w649:errorcluster)  [unwired: 1 in, 1 out]
                            n220 = call <vilib>:"General Error Handler.vi"("type of dialog (OK msg:1)"=1, "error in (no error)"=w649) -> ()  [unwired: 9 in, 5 out]
                          }
                        }
                        n221 = Number To Decimal String(number="Channel") -> (decimal integer string=w606:string)  [unwired: 1 in]
                      }
                      frame #4 {
                        n222 = call "Start.vi"("GPIB Address"=w662) -> ()  [unwired: 9 in]
                      }
                      frame #5 {
                        # "Wait for Scan to Finish"
                        n223 = for {
                          N: 1 -> [_]
                          tunnel: w667 -> [w669]
                          n224 = while {
                            tunnel: w669 -> [w670]
                            stop <- w672 stop-if-true
                            n225 = call "ScanDone.vi"("Wait (ms)"=1000, "GPIB Address"=w670) -> ("Scan Finished?"=w672:bool)
                          }
                        }
                      }
                      frame #6 {
                        w681 = 0
                        w689 = "\r\n"
                        n226 = call "Read Data.vi"("Channel Number"=0, "GPIB Address"=w710, "Number of Datapoints"=1) -> ("Data"=w711:i32[])
                        n227 = Index Array(array=w711, index=0) -> (element=w678:i32)
                        "Counts" <- w678
                        n228 = local read "Integrating time \nin 10^-7 sec"() -> (w687:dbl)
                        n229 = Replace Array Subset(array=w677, new element #1=w678, index (row) #1=w676, index (col) #1=w679, new element #2=w680, index (row) #2=w676, index (col) #2=w681, new element #3=w682, index (row) #3=w681, index (col) #3=w679) -> (w675:T6)
                        n230 = Array To Spreadsheet String(delimiter (Tab)=",", array=w675, 3:"%f" ("format string")) -> (spreadsheet string=w688:string)
                        n231 = local read "Blaze angle"() -> (w705:dbl)
                        n232 = local read "Grating #"() -> (w704:dbl)
                        n233 = Multiply(x=w687, y=1e-07) -> (x*y=w686:dbl)
                        n234 = Get Date/Time In Seconds() -> (seconds since 1Jan1904=w699:timestamp)
                        n235 = Format Date/Time String(time format string (%c)="%Y-%b-%d %H:%M:%S", seconds (now)=w699) -> (date/time string=w700:string)  [unwired: 1 in]
                        n236 = Number To Decimal String(number=w686) -> (decimal integer string=w701:string)  [unwired: 1 in]
                        n237 = Number To Decimal String(number=w704) -> (decimal integer string=w702:string)  [unwired: 1 in]
                        n238 = Number To Decimal String(number=w705) -> (decimal integer string=w690:string)  [unwired: 1 in]
                        n239 = call <vilib>:"Space Constant.vi"() -> ("String"=w703:string)
                        n240 = Open/Create/Replace File(file path (use dialog)="Data File Path", operation (0:open)=T5."replace or create") -> (refnum out=w709:refnum<file>)  [unwired: 4 in, 2 out]
                        n241 = Concatenate Strings(w689, "Data was taken on ", w700, w689, "Integration Time is ", w701, w703, "s", w689, "Monochromator gratng # ", w702, "; ", "blazed for ", w690, w703, "nm", w689, w689, w689, w688) -> (w684:string)
                        n242 = Write to Text File(file (use dialog)=w709, text=w684) -> (refnum out=w674:refnum<file>)  [unwired: 2 in, 2 out]
                        n243 = Flush File(refnum=w674) -> (refnum out=w673:refnum<file>)  [unwired: 1 in, 1 out]
                        n244 = Close File(refnum=w673) -> ()  [unwired: 1 in, 2 out]
                      }
                    }
                    n245 = Build Array (concatenate)(w551, w549) -> (w550:dbl[])
                    n246 = Bundle(w553, w550) -> (w548:cluster{dbl[], dbl[]})  [unwired: 1 in]
                    "Spectrum" <- w548
                    n247 = Unbundle(w548) -> (w547:dbl[], w552:dbl[])
                  }
                }
                frame #1 {
                  n248 = Array Size(array="Array") -> (size(s)=w717:i32)
                  n249 = flat-sequence {
                    tunnel: w715 -> [w724]
                    tunnel: "Array" -> [w723]
                    tunnel: w717 -> [w722]
                    tunnel: [w720] -> w718
                    frame #0 {
                      n250 = for {
                        N: w722 -> [_]
                        tunnel: w723 -> [w735]
                        tunnel: w724 -> [w730]
                        shift-right: [w725] -> w720
                        shift-left: dbl[] [] -> [w726]
                        i -> [w728]
                        n251 = local read "Scan from"() -> (w733:i32)
                        n252 = Index Array(array=w735, index=w728) -> (element=w734:dbl)
                        n253 = local read "Step size"() -> (w731:dbl)
                        n254 = Subtract(x=w734, y=w733) -> (x-y=w732:dbl)
                        n255 = Divide(x=w732, y=w731) -> (x/y=w729:dbl)
                        n256 = Index Array(array=w730, index=w729) -> (element=w727:dbl)
                        n257 = Insert Into Array(array=w726, index=w728, new element=w727) -> (w725:dbl[])
                      }
                    }
                  }
                }
              }
              n258 = local read "Scan from"() -> (w431:i32)
              n259 = local read "Step size"() -> (w429:dbl)
              n260 = To Time Stamp(1:w431) -> (0:w430:timestamp)
              n261 = Bundle By Name("Y"=w435, "t0"=w430, "dt"=w429) -> (w432:waveform(dbl))  [unwired: 1 in]
              n262 = Build Array (concatenate)(w434, w432) -> (w433:waveform(dbl)[])
              "Waveform Graph" <- w433
              n263 = for {
                N: w419 -> [_]
                tunnel: [w475] -> w427
                tunnel: w425 -> [w474]
                tunnel: w422 -> [w472]
                tunnel: [w471] -> w421
                tunnel: w420 -> [w473]
                tunnel: [w468] -> w418 mode=indexing
                i -> [w470]
                n264 = Build Array (concatenate)(w473, w472) -> (w471:dbl[][])
                n265 = Index Array(array=w472, index=w470) -> ()  [unwired: 1 out]
                n266 = Index Array(array=w471, index (col)=w470) -> (element=w469:dbl[])  [unwired: 1 in]
                n267 = Bundle(w474, w469) -> (w468:cluster{dbl[], dbl[]})  [unwired: 1 in]
                n268 = Unbundle(w468) -> (w475:dbl[])  [unwired: 1 out]
              }
              "Decay" <- w418
              "Current Point" <- w415
            }
            n269 = property on="Decay" class="XYGraph (strict)"("XScale.Increment"=w355, "XScale.Maximum"=w385, "XScale.Minimum"=w354) -> ()  [unwired: 2 in, 2 out]
            n270 = Build Array (concatenate)(0, w398) -> ()  [unwired: 1 out]
          }
        }
      }
    }
  }
  n271 = call "Configure.vi"("Dwell Time (s)"="Time between measurements\n at one point (s)/Dwell Time", "Channel T Input"="Trigger mode", "Channel B Input"="Channel B Input", "Channel A Input"="Channel A Input", "Integrating time, 10^-7 sec"="Integrating time \nin 10^-7 sec", "gate mode (CW:0)"="gate mode (CW:0)", "Scan End Mode"=FALSE, "Number of Periods"="Number of Measurements\n to take at one point/ Number of Periods", "Count Mode"="Count Mode", "GPIB Address"="GPIB address") -> ()
  "Mono port" <- w2
  "Time delay" <- w1
